vi "MoveIncSingle.vi"(5 "distance":dbl, 7 "speed":dbl min=0.0, 8 "error in (no error)":errorcluster, 9 "taskId":i32(ring) items=["TLibrary", "T01", "T02", "T03", "T04", "T05", "T06", "T07", "T08", "T09", "T10", "T11", "T12", "T13", "T14", "T15", "T16", "T17", "T18", "T19", "T20", "T21", "T22", "T23", "T24", "T25", "T26", "T27", "T28", "T29", "T30", "T31"], 10 "axis name":string, 11 "controller in":refnum<k24>) -> (0 "error out":errorcluster, 3 "controller out":refnum<k24>)   [LabVIEW 2018, in "Aerotech.lvlib"]
uses:
  Aerotech.lvlib
  C:/Program Files (x86)/Aerotech/A3200/LabVIEW/2010/Bin/Aerotech.A3200.dll
  Program Files (x86)/Aerotech/A3200/LabVIEW/2010/Bin/Aerotech.A3200.dll
  C:/Users/HEP/Documents/GitHub/UCSB-Gantry-HEP-2018/Drivers/Aerotech A3200/Bin/Aerotech.A3200.LabVIEW.dll
  UCSB-Gantry-HEP-2018/Drivers/Aerotech A3200/Bin/Aerotech.A3200.LabVIEW.dll
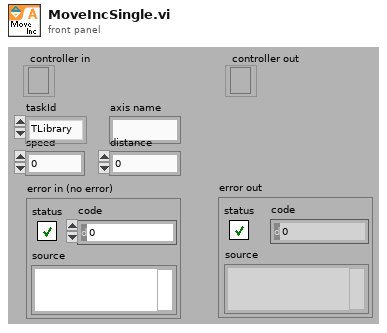
[diagram p1: front panel]
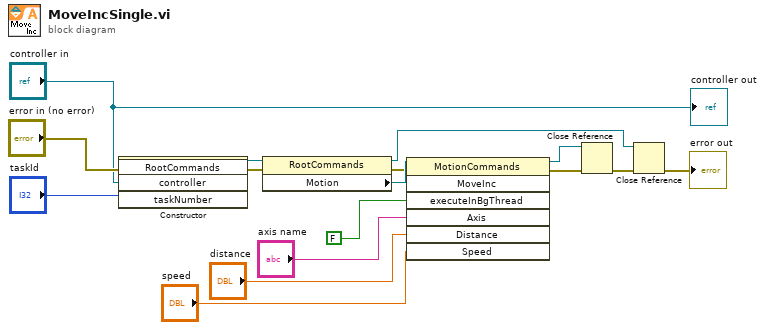
[diagram p0: block diagram]
diagram:
  n1 = constructor class="RootCommands"(error in="error in (no error)", "controller"="controller in", "taskNumber"="taskId") -> (reference out=w10:refnum<k24>, error out=w9:errorcluster)  [unwired: 2 in, 3 out]
  n2 = property class="RootCommands"(reference=w10, error in=w9) -> (reference out=w5:refnum<k24>, error out=w11:errorcluster, "Motion"=w12:refnum<k24>)
  n3 = invoke class="MotionCommands" method="MoveInc"(reference=w12, error in=w11, "executeInBgThread"=FALSE, "Axis"="axis name", "Distance"="distance", "Speed"="speed") -> (reference out=w7:refnum<k24>, error out=w8:errorcluster)  [unwired: 1 in, 5 out]
  n4 = Close Reference(reference=w7, error in (no error)=w8) -> (error out=w6:errorcluster)
  n5 = Close Reference(reference=w5, error in (no error)=w6) -> (error out=→"error out":errorcluster)
  "controller out" <- "controller in"
